vi "2017-03-23 TTTR Simple Test.vi"() -> ()   [LabVIEW 2016]
panel:
  out "Counts After":dbl
  out "Counts":dbl
  out "FiFo Overrun":bool
  out "OK":bool
  in  "Path":path=path "C:/Users/WilsonLab1/Desktop/test"
  out "Initialization Status":string
  out "Serial":string
  out "DLL Version":string
  out "DevIdx":dbl
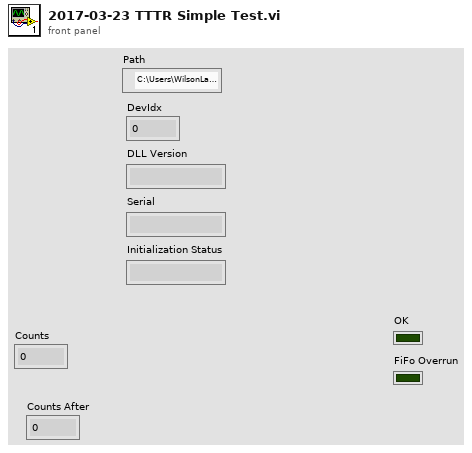
[diagram p1: front panel]
types:
  T1 = enum16{"open", "replace", "create", "open or create", "replace or create", "replace or create with confirmation"}
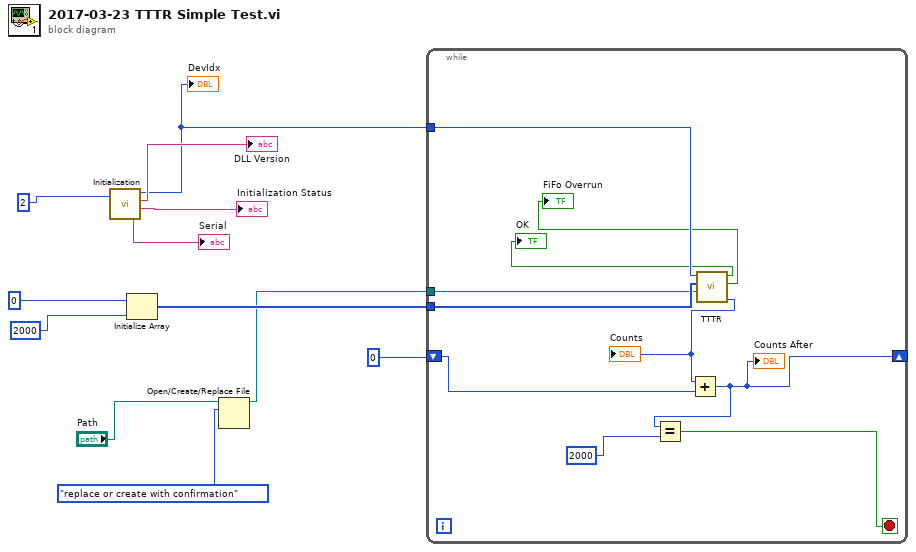
[diagram p0: block diagram]
diagram:
  n1 = call "Initialization.vi"("Mode"=2) -> ("Deviceindex"=w4:i32, "DLL Version"=→"DLL Version":string, "Initialization Status"=→"Initialization Status":string, "Serial[8]"=→"Serial":string)  [unwired: 1 out]
  "DevIdx" <- w4
  n2 = Initialize Array(0, 2000) -> (w3:i32[])
  n3 = Open/Create/Replace File(file path (use dialog)="Path", operation (0:open)=T1."replace or create with confirmation") -> (refnum out=w2:refnum<file>)  [unwired: 4 in, 2 out]
  n4 = while {
    tunnel: w4 -> [w22]
    tunnel: w3 -> [w21]
    tunnel: w2 -> [w20]
    shift-right: [w15] -> _
    shift-left: 0 -> [w17]
    stop <- w13 stop-if-true
    n5 = call "TTTR.vi"("file refnum"=w20, "Array"=w21, "DeviceIndex"=w22) -> ("count"=w16:i32, "FiFoOverrun"=→"FiFo Overrun":bool, "OK"=→"OK":bool)  [unwired: 1 in, 1 out]
    "Counts" <- w16
    n6 = Add(x=w16, y=w17) -> (x+y=w15:i32)
    "Counts After" <- w15
    n7 = Equal?(x=w15, y=2000) -> (x = y?=w13:bool)
  }
